vi "HQ Main.vi"() -> ()   [LabVIEW 2017]
uses:
  Type Defs/PodHealth.ctl
  Type Defs/PodStates.ctl
  Type Defs/PodState.ctl
panel:
  in  "FLaser Select":bool
  in  "SLaser Select":bool
  out "Pod State":T1
  out "Pusher Attached":bool
  in  "Phase":T2={"Pre-Flight Tests"=FALSE, "Ready"=FALSE, "Accelerate"=TRUE, "Coast"=FALSE, "Brake"=FALSE, "Post-Flight"=FALSE}
  in  "Detail Window":T3(tab)
  in  "Reset Sensors":bool
  in  "Vent":bool
  in  "Brake Boost":bool
  in  "Brake Open":bool
  in  "Sensor Power":bool
  in  "Activate Pneumatics":bool
  in  "Friction Brake":bool
  in  "Mag Brake":bool
  in  "Levitation":bool
  in  "Reset Laser Count":bool
  out "Acceleration (m/s^2)":dbl(graph)
  out "Velocity (m/s)":dbl(graph)
  out "Position":T4(graph)
  out "Pressure":T4(graph)
  out "Levitation Gap (mm)":T5(graph)
  out "Battery Monitor":cluster{"Voltage (Total)":dbl, "Power":dbl}(graph)={"Voltage (Total)"=11.91201, "Power"=9.516504789}
  in  "Laser Debounce Count":u8=10
  in  "Distance Between Tube Stripes (m)":dbl=30.49
  in  "Run ToF Calibration":bool=TRUE
  in  "Send Non-Critical Data":bool=TRUE
  in  "Velocity":dbl
  out "AutoSequence":bool
  out "Applying Brake State":bool
  in  "Ignore Rip Cord":bool
  out "Rip Cord Out?":bool
  in  "Timer Limit (s)":dbl
  in  "Stripe Count Limit":dbl
  out "Timer (s)":dbl
  out "Stripe Count":dbl
  in  "IMPORTANT - Enter Team ID":dbl
  in  "Mag Brake Setting":bool
  in  "Friction Brake Setting":bool
  in  "Brake Boost Setting":bool
  in  "Stop":bool
  out "Battery Current":dbl(knob)=9.144776890538314 scale=0.0..5.0
  out "Battery Voltage":dbl(knob)=11.942438656676648 scale=11.0..12.0
  out "Batt. Temp":dbl(slide)=81.63265306122449 scale=0.0..100.0
  out "Gap 4":u8(slide)=11 scale=0.0..100.0
  out "Gap 3":u8(slide)=10 scale=0.0..200.0
  out "Gap 2":u8(slide)=12 scale=0.0..100.0
  out "Gap 1":u8(slide)=13 scale=0.0..100.0
  out "Track Position":dbl(slide)=438.0053908355795 scale=0.0..1600.0
  out "Pod Health":T6={"Overall Pod Health"=TRUE, "Power"={"Power"=TRUE, "Friction Brakes"=TRUE, "Magnetic Brakes"=TRUE, "Primary Battery"=TRUE, "Backup Battery"=TRUE}, "Pressure"={"Pressure"=TRUE, "HP"=TRUE, "MP "=TRUE, "LP"=TRUE}, "Position"={"Position"=TRUE, "Maglock"=TRUE, "Levitation (ToF)"=TRUE}}
  # "TBD kick off calibration on ToF"
  # "100ft/30.48m - default"
  # "How many low detections \ndo we need before we \nrecognize a rising edge\n10 is safe, >3 is risky\nmax speed at 3 is 170mph"
  # "default 0 - so issue is obvious"
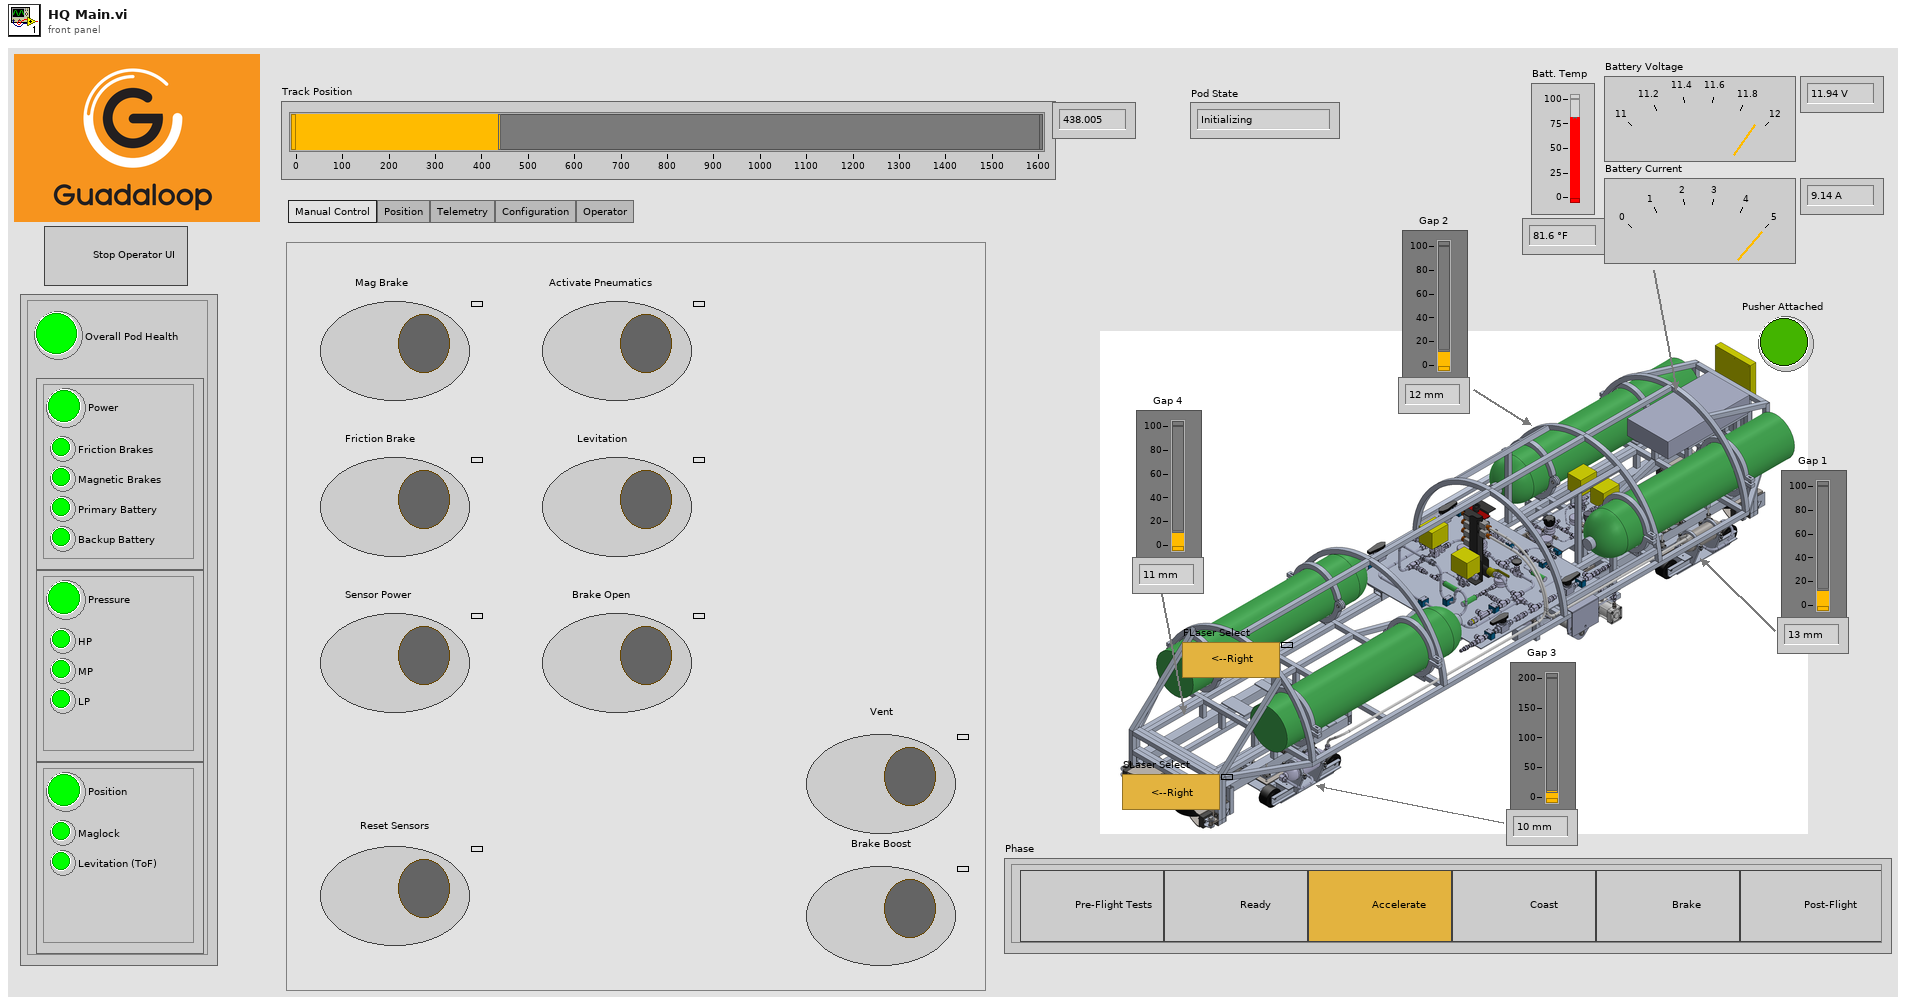
[diagram p1: front panel]
types:
  T1 = typedef "PodState.ctl" = enum16{"Initializing", "Pre-flight Testing", "Ready", "Pushing", "Coast", "Braking", "Post-flight", "Fault"}
  T2 = typedef "PodStates.ctl" = cluster{"Pre-Flight Tests":bool, "Ready":bool, "Accelerate":bool, "Coast":bool, "Brake":bool, "Post-Flight":bool}
  T3 = enum32{"Manual Control", "Position", "Telemetry", "Configuration", "Operator"}
  T4 = cluster{"Double":dbl, "Double":dbl, "Double":dbl, "Double":dbl}
  T5 = cluster{"UInt8":u8, "UInt8":u8, "UInt8":u8, "UInt8":u8}
  T6 = typedef "PodHealth.ctl" = cluster{"Overall Pod Health":bool, "Power":cluster{"Power":bool, "Friction Brakes":bool, "Magnetic Brakes":bool, "Primary Battery":bool, "Backup Battery":bool}, "Pressure":cluster{"Pressure":bool, "HP":bool, "MP ":bool, "LP":bool}, "Position":cluster{"Position":bool, "Maglock":bool, "Levitation (ToF)":bool}}
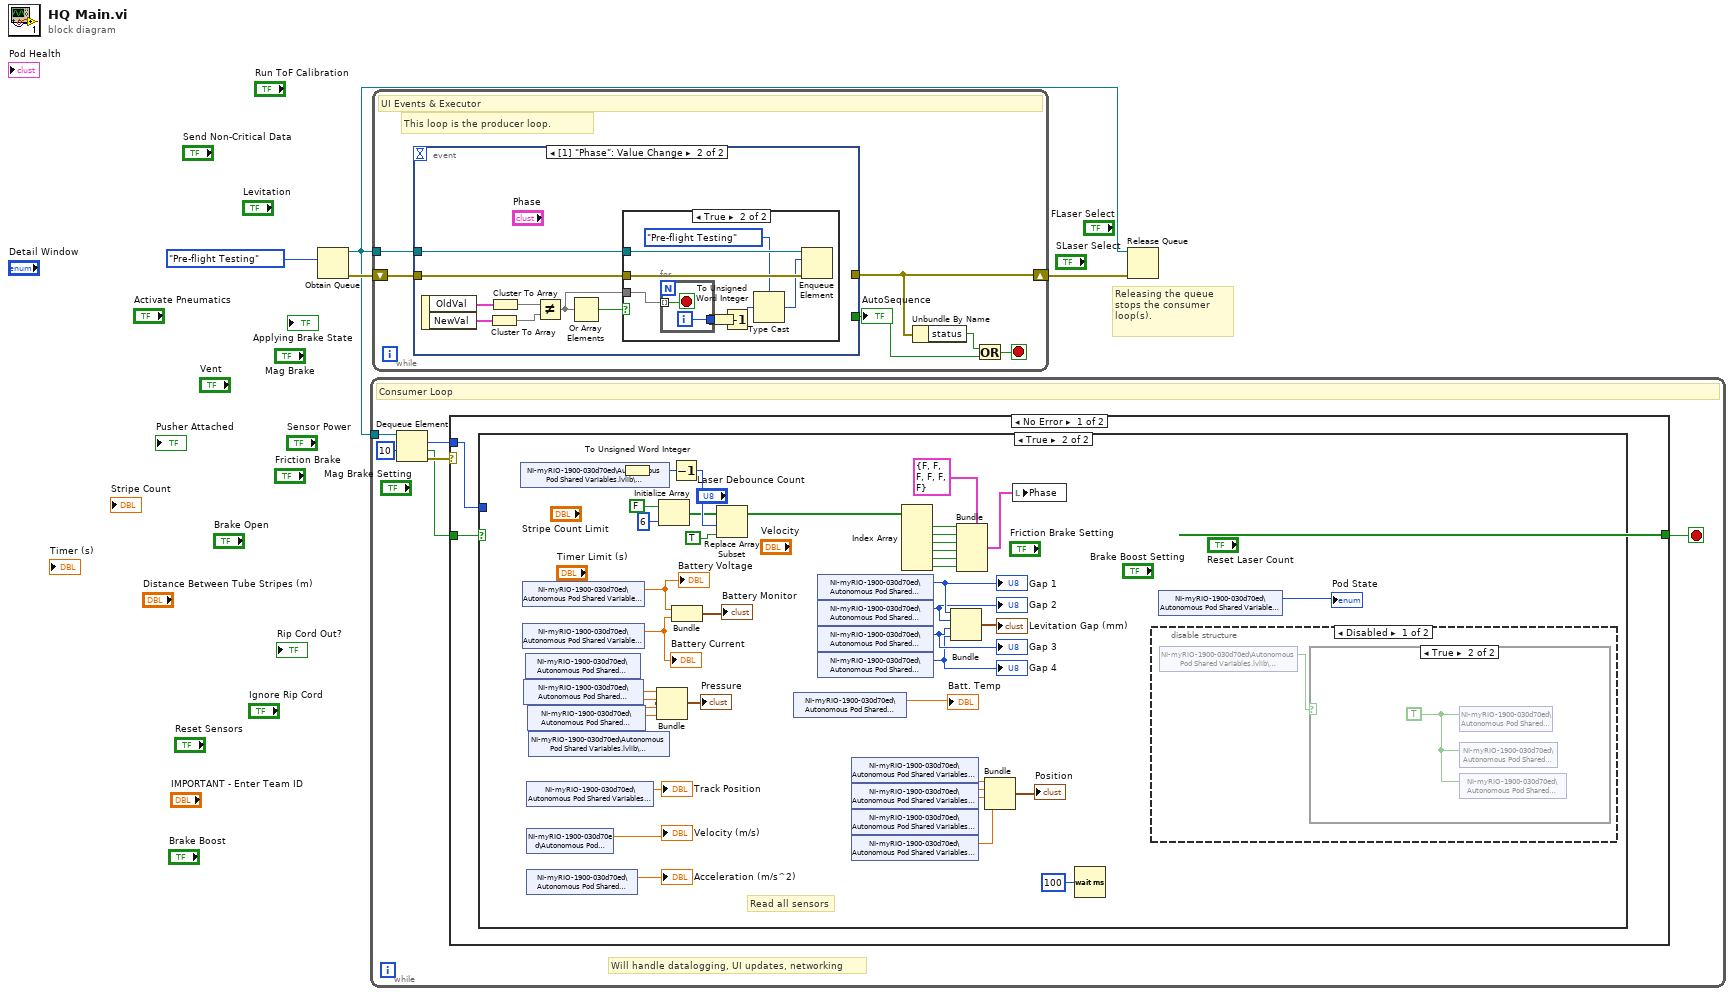
[diagram p0: block diagram]
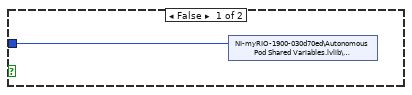
[diagram p2: hidden frame]
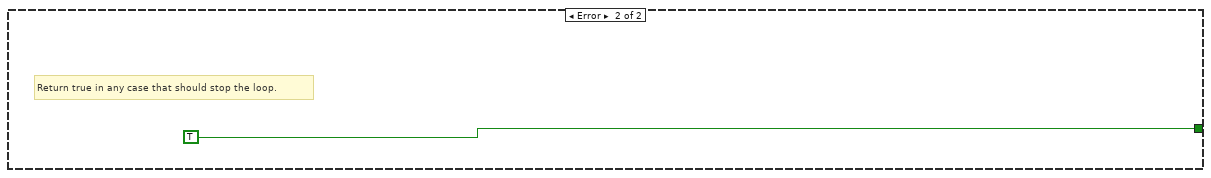
[diagram p5: hidden frame]
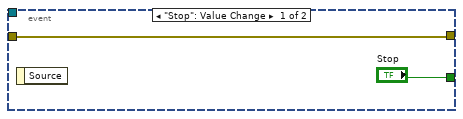
[diagram p6: hidden frame]
diagram:
  # "Releasing the queue stops the consumer loop(s)."
  n1 = Obtain Queue(element data type=PodState."Pre-flight Testing" ("Pod States")) -> (queue out=w2:refnum<queue>, error out=w4:errorcluster)  [unwired: 4 in, 1 out]
  n2 = while {
    tunnel: w2 -> [w10]
    stop <- w7 stop-if-true
    # "Will handle datalogging, UI updates, networking"
    # "Consumer Loop"
    n3 = Dequeue Element(queue=w10, timeout in ms (-1)=10) -> (element=w8:T1, timed out?=w5:bool, error out=w9:errorcluster)  [unwired: 1 in, 1 out]
    n4 = case shown="No Error" w9 {
      tunnel: w8 -> [w11 _]
      tunnel: [_ TRUE] -> w7
      tunnel: w5 -> [w12 _]
      frame No Error {
        n5 = case shown="True" w12 {
          tunnel: w11 -> [w13 _]
          frame False {
            n6 = shared-variable "NI-myRIO-1900-030d70ed\\Autonomous Pod Shared Variables.lvlib\\PodStateCommand"(w13) -> ()  [unwired: 1 in, 1 out]
          }
          frame True {
            # "Read all sensors"
            n7 = shared-variable "NI-myRIO-1900-030d70ed\\Autonomous Pod Shared Variables.lvlib\\PodStateCommand"() -> (w15:T1)  [unwired: 1 in, 1 out]
            n8 = shared-variable "NI-myRIO-1900-030d70ed\\Autonomous Pod Shared Variables.lvlib\\BatteryVoltage"() -> (w30:dbl)  [unwired: 1 in, 1 out]
            "Battery Voltage" <- w30
            n9 = shared-variable "NI-myRIO-1900-030d70ed\\Autonomous Pod Shared Variables.lvlib\\BatteryCurrent"() -> (w29:dbl)  [unwired: 1 in, 1 out]
            "Battery Current" <- w29
            n10 = shared-variable "NI-myRIO-1900-030d70ed\\Autonomous Pod Shared Variables.lvlib\\UtilityPressure"() -> (w36:dbl)  [unwired: 1 in, 1 out]
            n11 = shared-variable "NI-myRIO-1900-030d70ed\\Autonomous Pod Shared Variables.lvlib\\HighPressure"() -> (w37:dbl)  [unwired: 1 in, 1 out]
            n12 = shared-variable "NI-myRIO-1900-030d70ed\\Autonomous Pod Shared Variables.lvlib\\PositionSLaser2"() -> (→"Track Position":dbl)  [unwired: 1 in, 1 out]
            n13 = shared-variable "NI-myRIO-1900-030d70ed\\Autonomous Pod Shared Variables.lvlib\\Velocity"() -> (→"Velocity (m/s)":dbl)  [unwired: 1 in, 1 out]
            n14 = shared-variable "NI-myRIO-1900-030d70ed\\Autonomous Pod Shared Variables.lvlib\\Acceleration"() -> (→"Acceleration (m/s^2)":dbl)  [unwired: 1 in, 1 out]
            n15 = shared-variable "NI-myRIO-1900-030d70ed\\Autonomous Pod Shared Variables.lvlib\\BrakePressure"() -> (w35:dbl)  [unwired: 1 in, 1 out]
            n16 = shared-variable "NI-myRIO-1900-030d70ed\\Autonomous Pod Shared Variables.lvlib\\LevitationPressure"() -> (w34:dbl)  [unwired: 1 in, 1 out]
            n17 = To Unsigned Word Integer(number=w15) -> (unsigned 16bit integer=w40:u16)
            n18 = Bundle("Double"=w37, "Double"=w36, "Double"=w35, "Double"=w34) -> (→"Pressure":T4)  [unwired: 1 in]
            n19 = Initialize Array(FALSE, 6 ("dimension size")) -> (w43:bool[])
            n20 = Decrement(x=w40) -> (x-1=w45:u16)
            n21 = Bundle("Double"=w30, "Double"=w29) -> (→"Battery Monitor":cluster{"Double":dbl, "Double":dbl})  [unwired: 1 in]
            n22 = Replace Array Subset(array=w43, new element=TRUE, index=w45) -> (w47:bool[])
            n23 = shared-variable "NI-myRIO-1900-030d70ed\\Autonomous Pod Shared Variables.lvlib\\BatteryTemp"() -> (→"Batt. Temp":dbl)  [unwired: 1 in, 1 out]
            n24 = shared-variable "NI-myRIO-1900-030d70ed\\Autonomous Pod Shared Variables.lvlib\\ToF1Distance"() -> (w28:u8)  [unwired: 1 in, 1 out]
            "Gap 1" <- w28
            n25 = shared-variable "NI-myRIO-1900-030d70ed\\Autonomous Pod Shared Variables.lvlib\\ToF2Distance"() -> (w27:u8)  [unwired: 1 in, 1 out]
            "Gap 2" <- w27
            n26 = shared-variable "NI-myRIO-1900-030d70ed\\Autonomous Pod Shared Variables.lvlib\\ToF3Distance"() -> (w26:u8)  [unwired: 1 in, 1 out]
            "Gap 3" <- w26
            n27 = shared-variable "NI-myRIO-1900-030d70ed\\Autonomous Pod Shared Variables.lvlib\\ToF4Distance"() -> (w25:u8)  [unwired: 1 in, 1 out]
            "Gap 4" <- w25
            n28 = shared-variable "NI-myRIO-1900-030d70ed\\Autonomous Pod Shared Variables.lvlib\\PositionFLaser1"() -> (w22:dbl)  [unwired: 1 in, 1 out]
            n29 = shared-variable "NI-myRIO-1900-030d70ed\\Autonomous Pod Shared Variables.lvlib\\PositionFLaser2"() -> (w21:dbl)  [unwired: 1 in, 1 out]
            n30 = shared-variable "NI-myRIO-1900-030d70ed\\Autonomous Pod Shared Variables.lvlib\\PositionSLaser1"() -> (w20:dbl)  [unwired: 1 in, 1 out]
            n31 = shared-variable "NI-myRIO-1900-030d70ed\\Autonomous Pod Shared Variables.lvlib\\PositionSLaser2"() -> (w19:dbl)  [unwired: 1 in, 1 out]
            n32 = Index Array(array=w47) -> (element #1=w48:bool, element #2=w49:bool, element #3=w50:bool, element #4=w51:bool, element #5=w52:bool, element #6=w53:bool)  [unwired: 6 in]
            n33 = Bundle("UInt8"=w28, "UInt8"=w27, "UInt8"=w26, "UInt8"=w25) -> (→"Levitation Gap (mm)":T5)  [unwired: 1 in]
            n34 = Bundle(cluster=T2 {"Pre-Flight Tests"=FALSE, "Ready"=FALSE, "Accelerate"=FALSE, "Coast"=FALSE, "Brake"=FALSE, "Post-Flight"=FALSE} ("Phase"), "Pre-Flight Tests"=w48, "Ready"=w49, "Accelerate"=w50, "Coast"=w51, "Brake"=w52, "Post-Flight"=w53) -> (w39:T2)
            n35 = Bundle("Double"=w22, "Double"=w21, "Double"=w20, "Double"=w19) -> (→"Position":T4)  [unwired: 1 in]
            n36 = local write "Phase"(w39) -> ()
            n37 = Wait (ms)(milliseconds to wait=u32 100) -> ()  [unwired: 1 out]
            n38 = disable-structure shown="Disabled" {
              frame Disabled {
                n39 = shared-variable "NI-myRIO-1900-030d70ed\\Autonomous Pod Shared Variables.lvlib\\AutoSequenceOn"() -> (w54:bool)  [unwired: 1 in, 1 out]
                n40 = case shown="True" w54 {
                  frame False {
                  }
                  frame True {
                    w55 = TRUE ("IgnoreRipCord(Temp)")
                    n41 = shared-variable "NI-myRIO-1900-030d70ed\\Autonomous Pod Shared Variables.lvlib\\FricBrake"(w55) -> ()  [unwired: 1 in, 1 out]
                    n42 = shared-variable "NI-myRIO-1900-030d70ed\\Autonomous Pod Shared Variables.lvlib\\MagBrake"(w55) -> ()  [unwired: 1 in, 1 out]
                    n43 = shared-variable "NI-myRIO-1900-030d70ed\\Autonomous Pod Shared Variables.lvlib\\3way1Open"(w55) -> ()  [unwired: 1 in, 1 out]
                  }
                }
              }
              frame Enabled {
              }
            }
            n44 = shared-variable "NI-myRIO-1900-030d70ed\\Autonomous Pod Shared Variables.lvlib\\PodStateStatus"() -> (→"Pod State":T1)  [unwired: 1 in, 1 out]
          }
        }
      }
      frame Error {
        # "Return true in any case that should stop the loop."
      }
    }
  }
  n45 = while {
    shift-right: [w58] -> w3
    shift-left: w4 -> [w61]
    tunnel: w2 -> [w62]
    stop <- w59 stop-if-true
    # "This loop is the producer loop."
    # "UI Events & Executor"
    n46 = event shown="[1] \"Phase\": Value Change" {
      selector: _ -> [_ _]
      dyn-events: _ -> [_ _]
      timeout: _ -> [_ _]
      tunnel: w62 -> [_ w71]
      tunnel: w61 -> [w64 w70]
      tunnel: [w64 _] -> w58
      tunnel: ["Stop" _] -> w60
      event "Stop": Value Change {
        n47 = event-data() -> ()  [unwired: 1 in, 1 out]
      }
      event Value Change {
        n48 = event-data() -> ("OldVal"=w72:T2, "NewVal"=w69:T2)  [unwired: 1 in]
        n49 = Cluster To Array(cluster=w69) -> (array=w67:bool[])
        n50 = Cluster To Array(cluster=w72) -> (array=w68:bool[])
        n51 = Not Equal?(x=w68, y=w67) -> (x != y?=w65:bool[])
        n52 = Or Array Elements(Boolean array=w65) -> (logical OR=w66:bool)
        n53 = case shown="True" w66 {
          tunnel: w71 -> [_ w80]
          tunnel: w70 -> [_ w79]
          tunnel: w65 -> [_ w78]
          frame False {
          }
          frame True {
            n54 = for {
              tunnel: w78 -> [w82] mode=indexing
              tunnel: [w81] -> w77
              i -> [w81]
              stop <- w82 stop-if-true
            }
            n55 = To Unsigned Word Integer(number=w77) -> (unsigned 16bit integer=w73:u16)
            n56 = Increment(x=w73) -> (x+1=w74:u16)
            n57 = Type Cast(type=PodState."Pre-flight Testing" ("Pod States"), x=w74) -> (*(type *) &x=w75:T1)
            n58 = Enqueue Element(queue=w80, element=w75, error in (no error)=w79) -> ()  [unwired: 1 in, 3 out]
          }
        }
      }
    }
    n59 = Unbundle By Name(w58) -> ("status"=w57:bool)
    n60 = Or(x=w57, y=w60) -> (x .or. y?=w59:bool)
  }
  n61 = Release Queue(queue=w2, error in (no error)=w3) -> ()  [unwired: 1 in, 3 out]
